vi "Read Task Composite Group.vi"(8 "error in (no error)":errorcluster, 11 "Composite Task in":refnum<class "Composite Task.lvclass">) -> (0 "error out":errorcluster, 2 "Composite Task Group":refnum<class "Task Ancestor.lvclass">[](array[class]), 3 "Composite Task out":refnum<class "Composite Task.lvclass">)   [LabVIEW 2024, in "Composite Task.lvclass"]
uses:
  Composite Task.lvclass
  Task Ancestor/Task Ancestor.lvclass
  Composite Task.lvclass/Composite Task.ctl
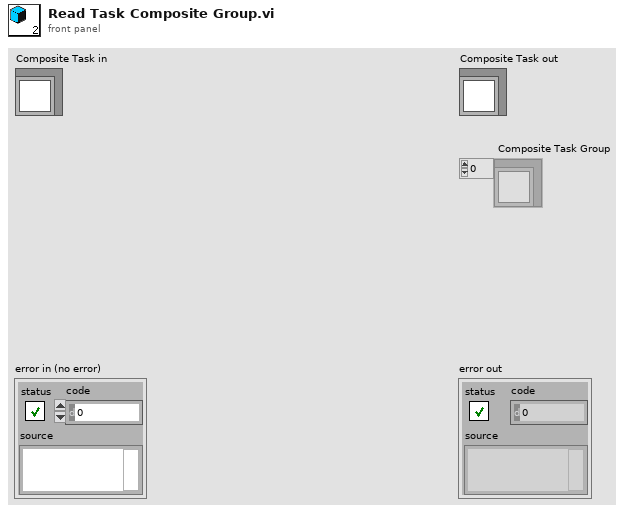
[diagram p1: front panel]
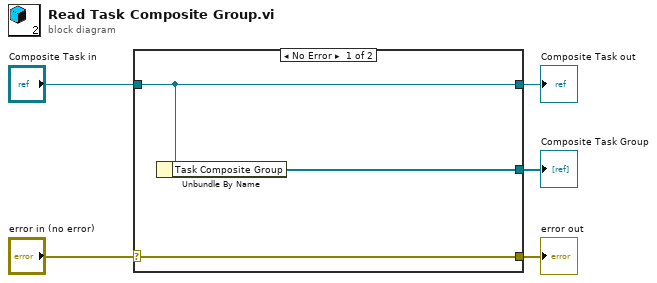
[diagram p0: block diagram]
diagram:
  n1 = case shown="No Error" "error in (no error)" {
    selector: "error in (no error)" -> [w8 w9]
    tunnel: [w8 w9] -> w4
    tunnel: [w7 w10] -> w2
    tunnel: "Composite Task in" -> [w7 w10]
    tunnel: [w6 _] -> w1
    frame No Error {
      n2 = Unbundle By Name(w7) -> ("Task Composite Group"=w6:refnum<class "Task Ancestor.lvclass">[])
    }
    frame Error {
    }
  }
  "error out" <- w4
  "Composite Task out" <- w2
  "Composite Task Group" <- w1
